vi "Test_Arduino_JIG.vi"() -> ()   [LabVIEW 2018, in "MB Relay.lvlib"]
uses:
  MB Relay.lvlib
  type defs/MB relays _InstrumentType.ctl
  type defs/FGV enum.ctl
  <vilib>/NI/Modbus Library/API/Master/Modbus Master.lvclass
panel:
  out "HoldingRegs 2":u16[](array[numeric])
  in  "read Registers":bool
  out "HoldingRegs":u16[](array[numeric])
  out "JIG trigger bit":bool
  in  "read jig trigger":bool
  in  "JIG reset":bool
  in  "jig reset":bool
  in  "VISA resource name":refnum<visa-resource-name>="COM16"
  in  "Open":bool
  in  "stop":bool
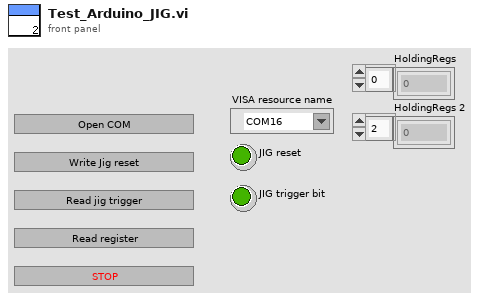
[diagram p1: front panel]
types:
  T1 = typedef "MB Relay.lvlib/FGV enum.ctl" = enum16{"Write", "Init FGV", "Read", "All OFF", "All ON"}
  T2 = typedef "MB Relay.lvlib/MB relays _InstrumentType.ctl" = enum16{"JIG_TRIGGER", "JIG_RESET", "Relay SelfTest", "counter", "demux1_10(x6)", "mux10_1(x6)", "mux6_1(3wires)", "MB_Relay_01(eMICs)", "SpareRelays(DPDT)", "Optos", "Inputs", "DMM I 0.5", "SpareRelays (SPDT)", "SC enable"}
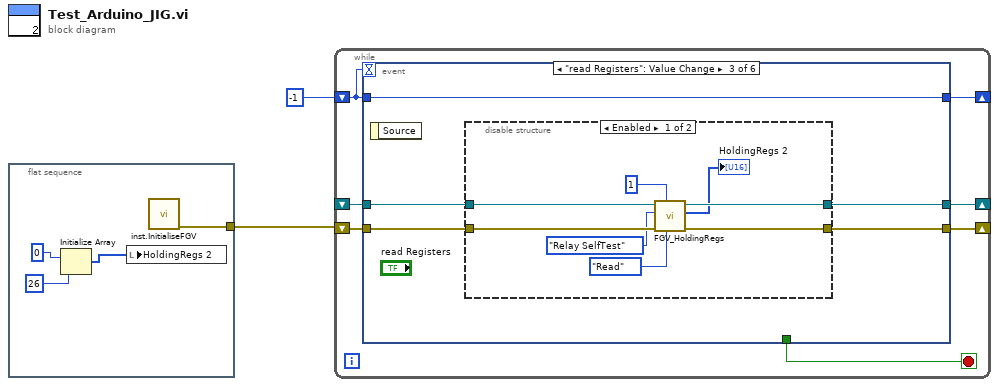
[diagram p0: block diagram]
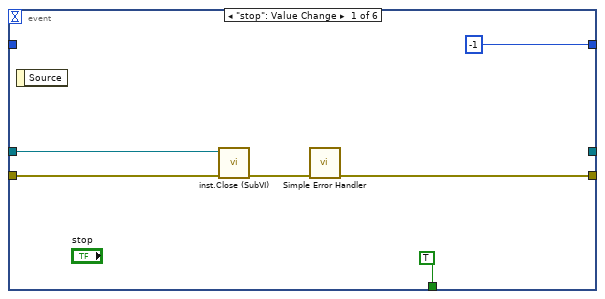
[diagram p2: hidden frame]
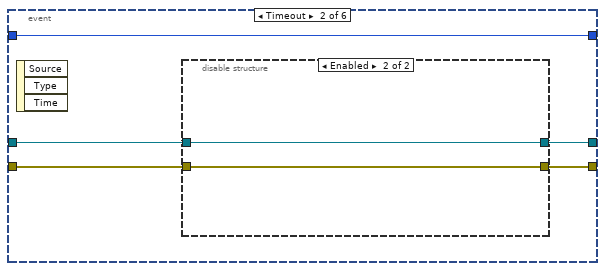
[diagram p3: hidden frame]
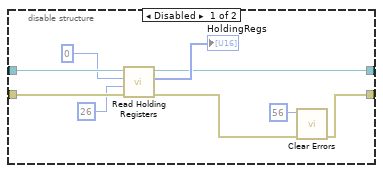
[diagram p4: hidden frame]
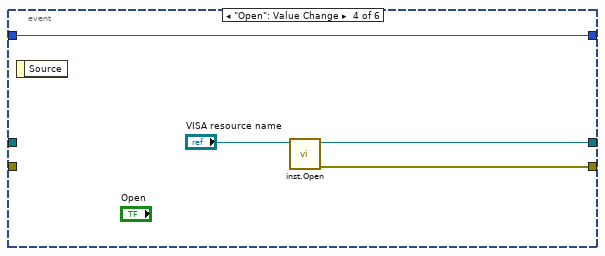
[diagram p6: hidden frame]
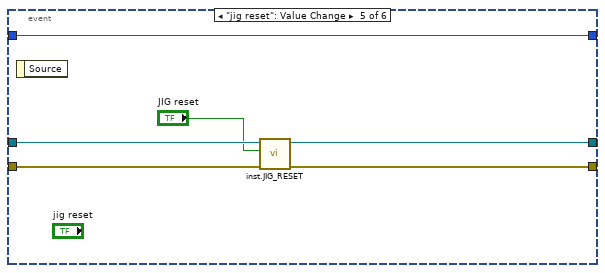
[diagram p7: hidden frame]
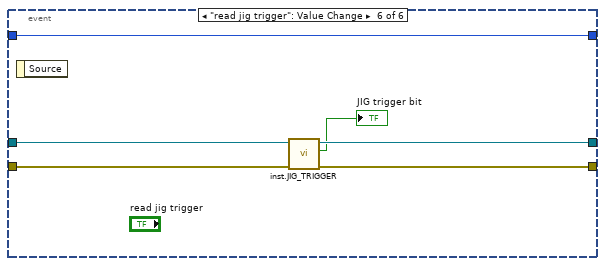
[diagram p8: hidden frame]
diagram:
  n1 = flat-sequence {
    tunnel: [w6] -> w1
    frame #0 {
      n2 = Initialize Array(u16 0, 26 ("dimension size")) -> (w3:u16[])
      n3 = local write "HoldingRegs 2"(w3) -> ()
      n4 = call "inst.InitialiseFGV.vi"() -> ("error out"=w6:errorcluster)  [unwired: 11 in]
    }
  }
  n5 = while {
    shift-right: [w12] -> _
    shift-left: _ -> [w10]
    shift-right: [w11] -> _
    shift-left: w1 -> [w9]
    shift-right: [w7] -> _
    shift-left: -1 -> [w8]
    stop <- w13 stop-if-true
    n6 = event shown="[2] \"read Registers\": Value Change" {
      selector: _ -> [_ _ _ _ _ _]
      dyn-events: _ -> [_ _ _ _ _ _]
      timeout: w8 -> [_ _ _ _ _ _]
      tunnel: [TRUE _ _ _ _ _] -> w13
      tunnel: [_ w22 w37 w53 w59 w63] -> w12
      tunnel: [w16 w20 w36 w52 w57 w64] -> w11
      tunnel: w10 -> [w17 w23 w39 _ w60 w66]
      tunnel: w9 -> [w15 w21 w38 _ w58 w65]
      tunnel: w8 -> [_ w24 w40 w51 w55 w61]
      tunnel: [-1 w24 w40 w51 w55 w61] -> w7
      event "stop": Value Change {
        n7 = event-data() -> ()  [unwired: 1 in, 1 out]
        n8 = call "inst.Close (SubVI).vi"("error in (no error)"=w15, "Modbus Master in"=w17) -> ("error out"=w19:errorcluster)  [unwired: 9 in]
        n9 = call <vilib>:"Simple Error Handler.vi"("error in (no error)"=w19) -> ("error out"=w16:errorcluster)  [unwired: 4 in, 4 out]
      }
      event Timeout {
        n10 = event-data() -> ()  [unwired: 1 in, 3 out]
        n11 = disable-structure shown="Enabled" {
          disable-tunnel: w23 -> [w33 w34]
          disable-tunnel: [w30 w34] -> w22
          disable-tunnel: w21 -> [w29 w35]
          disable-tunnel: [w25 w35] -> w20
          frame Disabled {
            n12 = call-dynamic "Read Holding Registers.vi"("error in"=w29, "number of inputs"=u16 26, "starting address"=u16 0, "Modbus master in"=w33) -> ("error out"=w26:errorcluster, "register values"=→"HoldingRegs":u16[], "Modbus master out"=w30:refnum<class "Modbus Master.lvclass">)  [unwired: 5 in]
            n13 = call <vilib>:"Clear Errors.vi"("error in (no error)"=w26, "specific error code to clear (0: all)"=56) -> ("error out"=w25:errorcluster)  [unwired: 4 in, 1 out]
          }
          frame Enabled {
          }
        }
      }
      event "read Registers": Value Change {
        n14 = event-data() -> ()  [unwired: 1 in, 1 out]
        n15 = disable-structure shown="Enabled" {
          disable-tunnel: w39 -> [w48 w49]
          disable-tunnel: [w45 w49] -> w37
          disable-tunnel: w38 -> [w47 w50]
          disable-tunnel: [w44 w50] -> w36
          frame Enabled {
            n16 = call "FGV_HoldingRegs.vi"("FGV_enum"=FGV_enum."Read", "unit ID"=u8 1, "error in (no error)"=w47, "Instruments"=MB_relays__InstrumentType."Relay SelfTest", "Modbus master in"=w48) -> ("error out"=w44:errorcluster, "HoldingRegs"=→"HoldingRegs 2":u16[], "Modbus master out"=w45:refnum<class "Modbus Master.lvclass">)  [unwired: 4 in]
          }
          frame Disabled {
          }
        }
      }
      event "Open": Value Change {
        n17 = event-data() -> ()  [unwired: 1 in, 1 out]
        n18 = call "inst.Open.vi"("VISA resource name"="VISA resource name") -> ("error out"=w52:errorcluster, "Modbus Master out"=w53:refnum<class "Modbus Master.lvclass">)  [unwired: 9 in]
      }
      event "jig reset": Value Change {
        n19 = event-data() -> ()  [unwired: 1 in, 1 out]
        n20 = call "inst.JIG_RESET.vi"("error in (no error)"=w58, "JIG reset"="JIG reset", "Modbus Master in"=w60) -> ("error out"=w57:errorcluster, "Modbus Master out"=w59:refnum<class "Modbus Master.lvclass">)  [unwired: 7 in]
      }
      event "read jig trigger": Value Change {
        n21 = event-data() -> ()  [unwired: 1 in, 1 out]
        n22 = call "inst.JIG_TRIGGER.vi"("error in (no error)"=w65, "Modbus master in"=w66) -> ("error out"=w64:errorcluster, "JIG_TRIGGER"=→"JIG trigger bit":bool, "Modbus master out"=w63:refnum<class "Modbus Master.lvclass">)  [unwired: 6 in, 1 out]
      }
    }
  }
